vi "PicoScope5000aExampleRapidBlockBulk.vi"() -> ()   [LabVIEW 2020]
panel:
  out "Channel B":T1(graph)
  in  "Channel B Settings 2":T2={"Enabled"=TRUE, "Coupling"=1, "Range"=6, "Analogue Offset"=0.0} {"Range" items=["10 mV", "20 mV", "50 mV", "100 mV", "200 mV", "500 mV", "1 V", "2 V", "5 V", "10 V", "20 V", "50 V ", "100 V"]; "Coupling" items=["AC", "DC"]}
  in  "Rapid Block Acquisition Settings":T3={"preTriggerSamples"=0, "postTriggerSamples"=1000, "timebase"=2, "Down-Sample Mode"=0, "Down Sample Ratio"=1, "Number of Captures"=10} {"Down Sample Ratio" min=1 step=1; "Down-Sample Mode" items=["None"=0, "Aggregate"=1, "Decimate"=2, "Average"=4]}
  out "Channel A":T1(graph)
  out "Device Info":T4
  out "Properties Panel":T5 {"Max Total Capture Time Available (sec)" format="%.3p"; "Sample Frequency" format="%.3p"; "Sample Rate" format="%.3p"; "Max Samples Available" format="%.3p"; "Total Capture Time (sec)" format="%.3p"}
  in  "Trigger Settings":T6={"Trigger Enabled"=FALSE, "Trigger Source"=enum."Channel A", "Trigger Threshold (volts)"=0.0, "Trigger Direction"=2, "Trigger Delay (samples)"=0, "Auto Trigger Time (ms)"=1000} {"Trigger Direction" items=["Rising"=2, "Falling"=3]}
  out "2-channel USB 3.0 device on non-USB 3.0 Port":bool=TRUE
  out "4-channel USB Powered":bool=TRUE
  in  "Serial Number":string
  in  "Use Serial Number":bool
  out "Number of Samples \nPer Capture":u32
  in  "Resolution":i32(ring)=1 items=["8-bit", "12-bit", "14-bit", "15-bit (max. 2 ch.)", "16-bit (max. 1 ch.)"]
  in  "Channel A Settings":T2={"Enabled"=TRUE, "Coupling"=1, "Range"=6, "Analogue Offset"=0.0} {"Range" items=["10 mV", "20 mV", "50 mV", "100 mV", "200 mV", "500 mV", "1 V", "2 V", "5 V", "10 V", "20 V", "50 V ", "100 V"]; "Coupling" items=["AC", "DC"]}
  out "Capture Complete":bool
  in  "Run":bool
  in  "Capture Index":i16 min=0
  in  "stop":bool
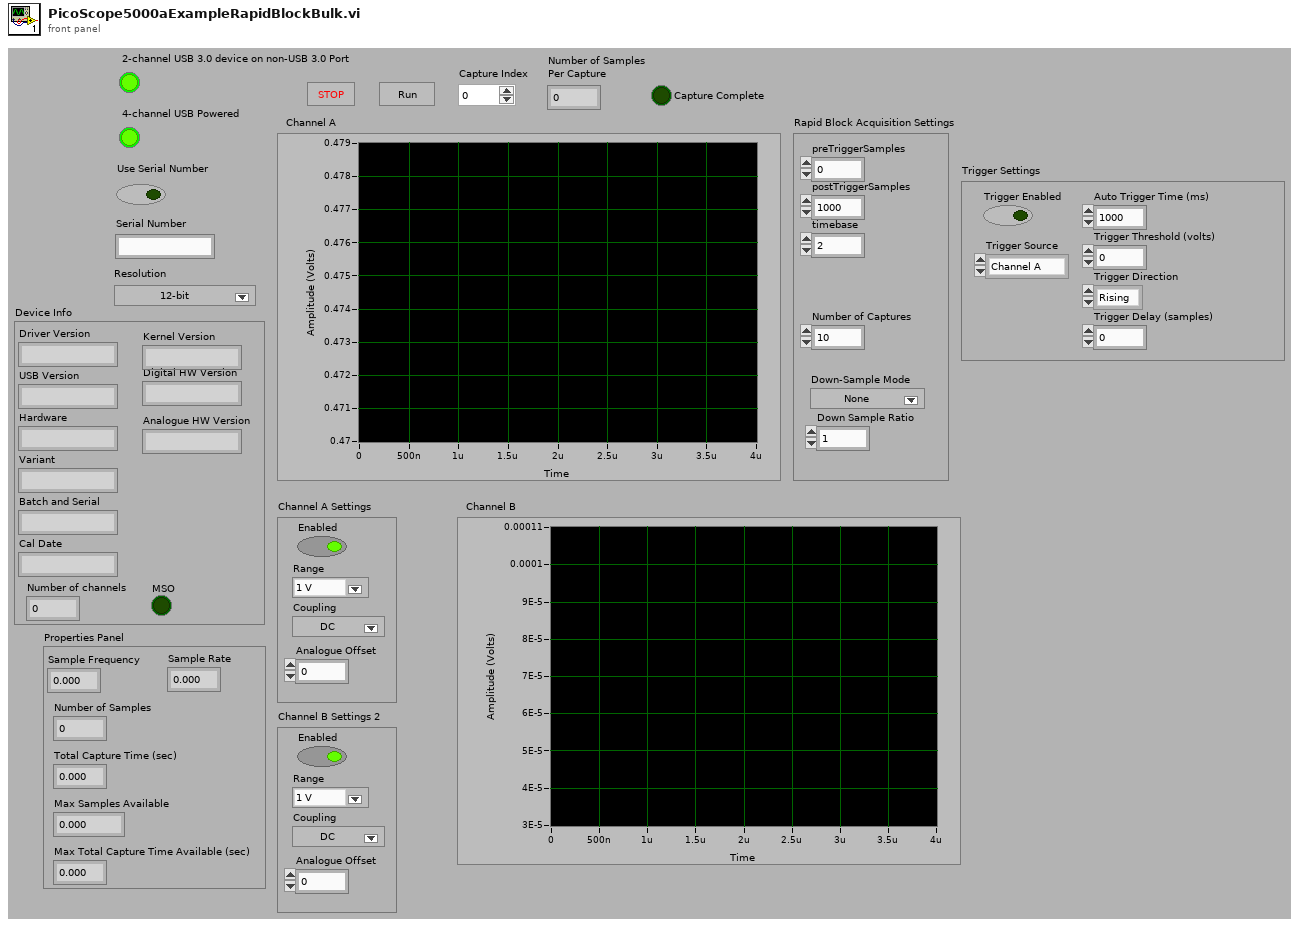
[diagram p1: front panel]
types:
  T1 = cluster{i32, "Sample Internal":sgl, "Data (Volts)":dbl[]}
  T2 = cluster{"Enabled":bool, "Coupling":i16, "Range":u16, "Analogue Offset":sgl}
  T3 = cluster{"preTriggerSamples":u32, "postTriggerSamples":u32, "timebase":u32, "Down-Sample Mode":i32, "Down Sample Ratio":u32, "Number of Captures":u32}
  T4 = cluster{"Driver Version":string, "USB Version":string, "Hardware":string, "Variant":string, "Batch and Serial":string, "Cal Date":string, "Kernel Version":string, "Digital HW Version":string, "Analogue HW Version":string, "MSO":bool, "Number of channels":i16}
  T5 = cluster{"Sample Frequency":sgl, "Sample Rate":sgl, "Max Samples Available":i32, "Number of Samples":u32, "Total Capture Time (sec) ":sgl, "Max Total Capture Time Available (sec)":sgl}
  T6 = cluster{"Trigger Enabled":bool, "Trigger Source":enum16{"Channel A", "Channel B", "Channel C", "Channel D", "Ext."}, "Trigger Threshold (volts)":dbl, "Trigger Direction":u16, "Trigger Delay (samples)":u32, "Auto Trigger Time (ms)":i16}
  T7 = cluster{"preTriggerSamples":u32, "postTriggerSamples":u32, "timebase":u32, "Down-Sample Mode":i32, "Down Sample Ratio":u32}
  T8 = cluster{i32, "Sample Rate":sgl, "Data (Volts)":dbl[]}
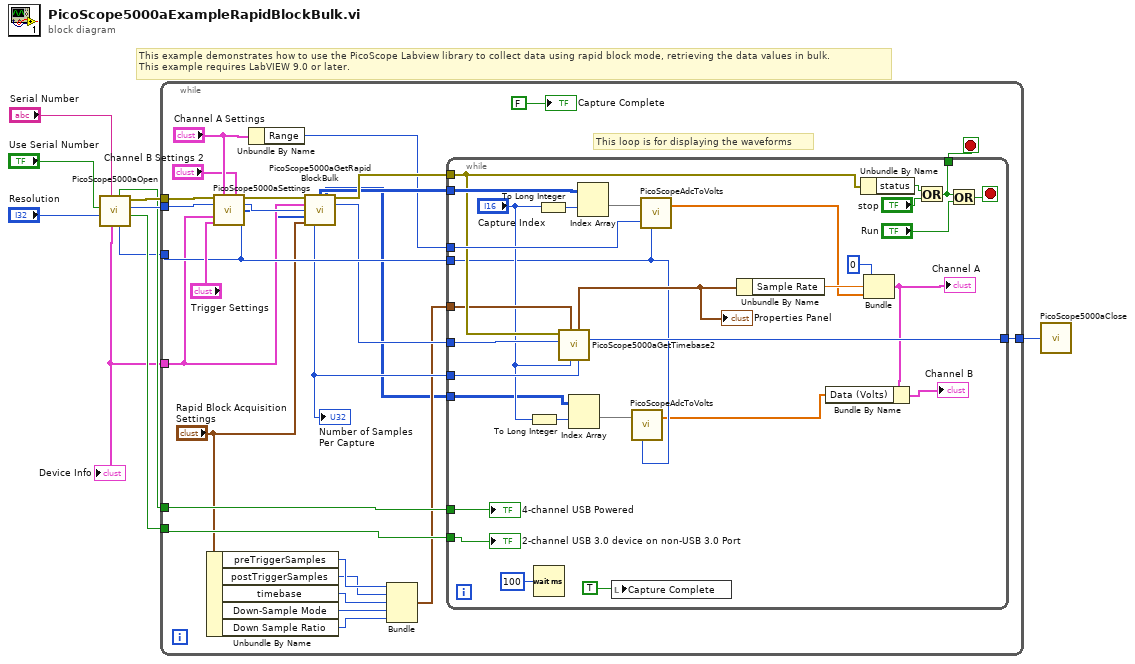
[diagram p0: block diagram]
diagram:
  # "This example demonstrates how to use the PicoScope Labview library to collect data using rapid block mode, retrieving the data values in bulk.\nThis example requires LabVIEW 9.0 or later."
  n1 = call "PicoScope5000aOpen.vi"("Serial Number"="Serial Number", "Resolution"="Resolution", "Use Serial Number"="Use Serial Number") -> ("USB Powered"=w7:bool, "handle"=w8:i16, "error out"=w9:errorcluster, "Max ADC value"=w2:i16, "USB 3.0 device on non-USB 3.0 Port"=w3:bool, "Device Info"=w1:T4)  [unwired: 3 in]
  "Device Info" <- w1
  n2 = while {
    tunnel: [w26] -> w10
    tunnel: w9 -> [w35]
    tunnel: w8 -> [w34]
    tunnel: w7 -> [w33]
    tunnel: w3 -> [w31]
    tunnel: w2 -> [w29]
    tunnel: w1 -> [w21]
    stop <- w38 stop-if-true
    # "This loop is for displaying the waveforms"
    n3 = Unbundle By Name("Rapid Block Acquisition Settings") -> ("preTriggerSamples"=w19:u32, "postTriggerSamples"=w18:u32, "timebase"=w16:u32, "Down-Sample Mode"=w15:i32, "Down Sample Ratio"=w14:u32)
    n4 = call "PicoScope5000aSettings.vi"("error in"=w35, "Channel A Settings"="Channel A Settings", "Channel B Settings"="Channel B Settings 2", "handle in"=w34, "Device Info"=w21, "Trigger Settings"="Trigger Settings", "Max ADC value"=w29) -> ("error out"=w25:errorcluster, "handle out"=w22:i16, "enabled array"=w13:i16[])  [unwired: 6 in]
    n5 = Unbundle By Name("Channel A Settings") -> ("Range"=w27:u16)
    n6 = call "PicoScope5000aGetRapidBlockBulk.vi"("error in"=w25, "Device Info"=w21, "handle in"=w22, "enabled array"=w13, "Rapid Block Acquisition Settings"="Rapid Block Acquisition Settings") -> ("Channel A Buffer"=w32:i16[][], "Channel B Buffer"=w11:i16[][], "error out"=w36:errorcluster, "handle out"=w23:i16, "Num samples"=w24:u32)  [unwired: 2 in, 4 out]
    "Number of Samples \nPer Capture" <- w24
    n7 = Bundle("preTriggerSamples"=w19, "postTriggerSamples"=w18, "timebase"=w16, "Down-Sample Mode"=w15, "Down Sample Ratio"=w14) -> (w20:T7)  [unwired: 1 in]
    n8 = while {
      tunnel: [w67] -> w38
      tunnel: w32 -> [w61]
      tunnel: w36 -> [w54]
      tunnel: w33 -> [w47]
      tunnel: w31 -> [w48]
      tunnel: w29 -> [w42]
      tunnel: w27 -> [w60]
      tunnel: [w53] -> w26
      tunnel: w24 -> [w52]
      tunnel: w23 -> [w51]
      tunnel: w20 -> [w49]
      tunnel: w11 -> [w43]
      stop <- w66 stop-if-true
      n9 = To Long Integer(number="Capture Index") -> (32bit integer=w46:i32)
      n10 = Wait (ms)(milliseconds to wait=u32 100) -> ()  [unwired: 1 out]
      n11 = To Long Integer(number="Capture Index") -> (32bit integer=w50:i32)
      n12 = call "PicoScope5000aGetTimebase2.vi"("Number of Samples"=w52, "Memory Segment"="Capture Index", "Acquisition Settings"=w49, "handle in"=w51, "error in (no error)"=w54) -> ("handle out"=w53:i16, "Properties Panel"=w55:T5)  [unwired: 4 in, 1 out]
      "Properties Panel" <- w55
      n13 = Index Array(array=w43, index (row)=w46) -> (element=w45:i16[])  [unwired: 1 in]
      n14 = Index Array(array=w61, index (row)=w50) -> (element=w59:i16[])  [unwired: 1 in]
      n15 = local write "Capture Complete"(TRUE ("Capture Complete")) -> ()
      n16 = call "PicoScopeAdcToVolts.vi"("Max_adc"=w42, "Data"=w45) -> ("Data (Volts)"=w40:dbl[])  [unwired: 1 in]
      n17 = call "PicoScopeAdcToVolts.vi"("Max_adc"=w42, "Range Index"=w60, "Data"=w59) -> ("Data (Volts)"=w56:dbl[])
      n18 = Unbundle By Name(w55) -> ("Sample Rate"=w57:sgl)
      n19 = Unbundle By Name(w54) -> ("status"=w62:bool)
      n20 = Bundle(0, "Sample Rate"=w57, "Data (Volts)"=w56) -> (w41:T8)  [unwired: 1 in]
      "Channel A" <- w41
      n21 = Bundle By Name(cluster=w41, "Data (Volts)"=w40) -> (→"Channel B":T8)
      n22 = Or(x=w62, y="stop") -> (x .or. y?=w67:bool)
      n23 = Or(x=w67, y="Run") -> (x .or. y?=w66:bool)
      "4-channel USB Powered" <- w48
      "2-channel USB 3.0 device on non-USB 3.0 Port" <- w47
    }
    "Capture Complete" <- FALSE ("Capture Complete")
  }
  n24 = call "PicoScope5000aClose.vi"("handle"=w10) -> ()
